vi "metres per second to mins per km.vi"(9 "Type":string, 10 "Moving Time (s)":dbl, 11 "Distance (m)":dbl) -> (1 "Type Out":string, 2 "Distance (km)":dbl, 3 "mins/km":dbl)   [LabVIEW 2020, in "Data Manager.lvclass"]
uses:
  Data Manager.lvclass
panel:
  out "m/s":dbl
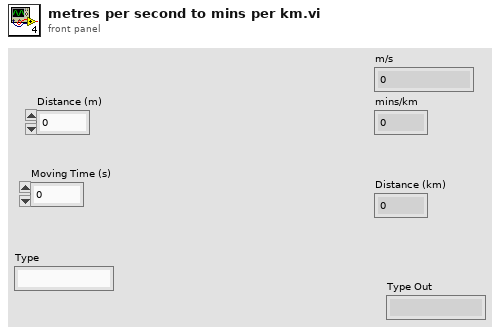
[diagram p1: front panel]
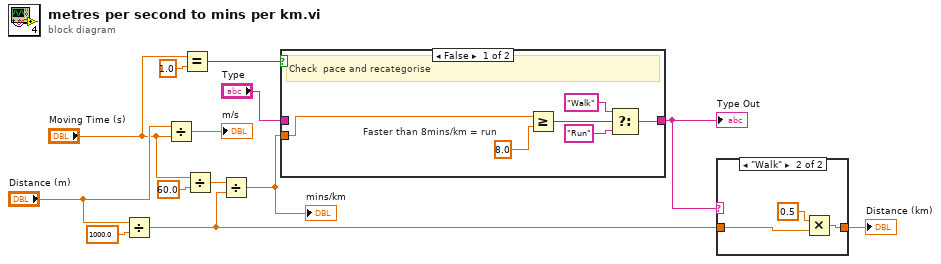
[diagram p0: block diagram]
diagram:
  n1 = Divide(x="Distance (m)", y=1000.0) -> (x/y=w2:dbl)
  n2 = Divide(x="Distance (m)", y="Moving Time (s)") -> (x/y=→"m/s":dbl)
  n3 = Equal?(x="Moving Time (s)", y=1.0) -> (x = y?=w6:bool)
  n4 = Divide(x="Moving Time (s)", y=60.0) -> (x/y=w9:dbl)
  n5 = Divide(x=w9, y=w2) -> (x/y=w1:dbl)
  "mins/km" <- w1
  n6 = case shown="False" w6 {
    tunnel: [w16 w20] -> w4
    tunnel: "Type" -> [_ w20]
    tunnel: w1 -> [w19 _]
    frame False {
      w18 = 8.0  # Faster than 8mins/km = run
      # "Check  pace and recategorise"
      n7 = Greater Or Equal?(x=w19, y=w18) -> (x >= y?=w17:bool)
      n8 = Select(t="Walk", s=w17, f="Run") -> (s? t:f=w16:string)
    }
    frame True {
      # "No Change"
    }
  }
  "Type Out" <- w4
  n9 = case shown="\"Walk\"" w4 {
    tunnel: [w21 w22] -> w3
    tunnel: w2 -> [w21 w24]
    frame Default {
    }
    frame "Walk" {
      n10 = Multiply(x=0.5, y=w24) -> (x*y=w22:dbl)
    }
  }
  "Distance (km)" <- w3
